vi "Configure Event Search (Serial Bus - SENT).vi"(6 "Slow Data (-1)":i32=-1, 7 "Slow ID (-1)":i32=-1, 8 "error in (no error)":errorcluster, 9 "Fast Data (0x)":string="0x", 10 "Search Operation (0: Fast Data)":i32(ring) items=["Fast Data", "Slow ID", "Slow ID and Data", "All CRC Errors", "Pulse Period Error"], 11 "VISA resource name":refnum<visa-resource-name>) -> (0 "error out":errorcluster, 3 "VISA resource name out":refnum<visa-resource-name>)   [LabVIEW 2023, in "Keysight-DSQx3014T.lvlib"]
doc: "Configures a search on a SENT serial decode signal.\n\n<b>Note:</b> SENT serial decode must be turned on and displayed in the Lister before running this VI."
uses:
  Keysight-DSQx3014T.lvlib
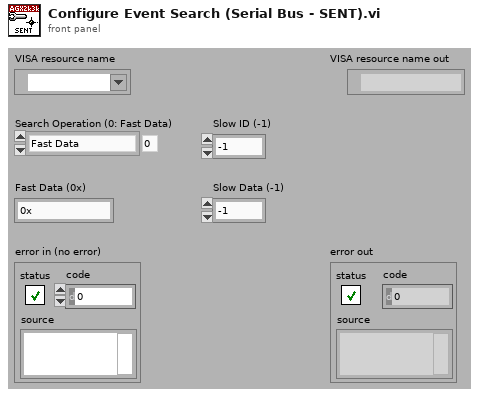
[diagram p1: front panel]
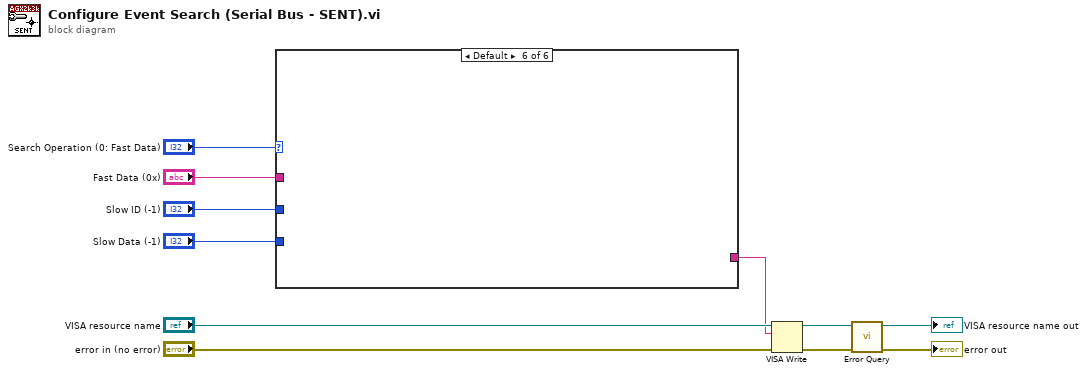
[diagram p0: block diagram]
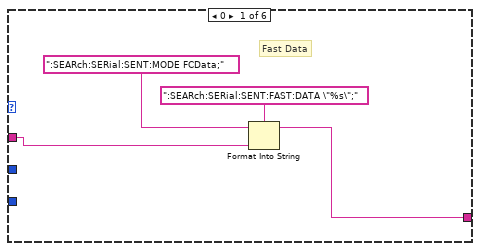
[diagram p2: hidden frame]
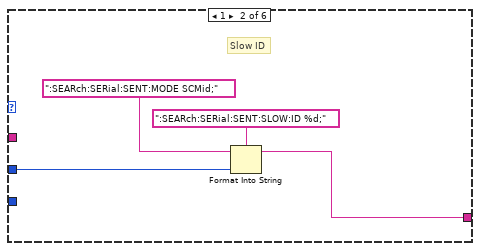
[diagram p3: hidden frame]
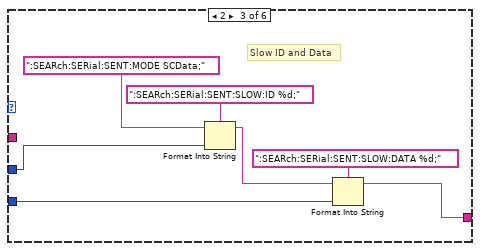
[diagram p4: hidden frame]
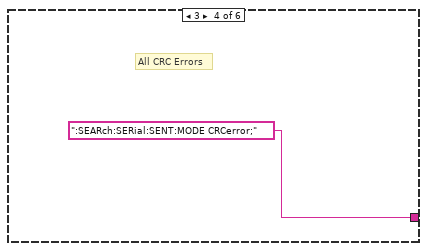
[diagram p5: hidden frame]
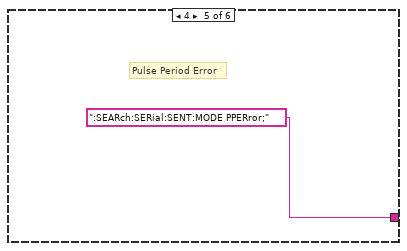
[diagram p6: hidden frame]
diagram:
  n1 = case shown="Default" "Search Operation (0: Fast Data)" {
    tunnel: "Fast Data (0x)" -> [w13 _ _ _ _ _]
    tunnel: [w12 w18 w23 ":SEARch:SERial:SENT:MODE CRCerror;" ":SEARch:SERial:SENT:MODE PPERror;" _] -> w7
    tunnel: "Slow ID (-1)" -> [_ w16 w22 _ _ _]
    tunnel: "Slow Data (-1)" -> [_ _ w20 _ _ _]
    frame 0 {
      # "Fast Data"
      n2 = Format Into String(format string=":SEARch:SERial:SENT:FAST:DATA \"%s\";", initial string=":SEARch:SERial:SENT:MODE FCData;", w13) -> (resulting string=w12:string)  [unwired: 1 in, 1 out]
    }
    frame 1 {
      # "Slow ID"
      n3 = Format Into String(format string=":SEARch:SERial:SENT:SLOW:ID %d;", initial string=":SEARch:SERial:SENT:MODE SCMid;", w16) -> (resulting string=w18:string)  [unwired: 1 in, 1 out]
    }
    frame 2 {
      # "Slow ID and Data"
      n4 = Format Into String(format string=":SEARch:SERial:SENT:SLOW:ID %d;", initial string=":SEARch:SERial:SENT:MODE SCData;", w22) -> (resulting string=w21:string)  [unwired: 1 in, 1 out]
      n5 = Format Into String(format string=":SEARch:SERial:SENT:SLOW:DATA %d;", initial string=w21, w20) -> (resulting string=w23:string)  [unwired: 1 in, 1 out]
    }
    frame 3 {
      # "All CRC Errors"
    }
    frame 4 {
      # "Pulse Period Error"
    }
    frame Default {
    }
  }
  n6 = VISA Write(VISA resource name="VISA resource name", write buffer=w7, error in (no error)="error in (no error)") -> (VISA resource name out=w4:refnum<visa-resource-name>, error out=w3:errorcluster)  [unwired: 1 out]
  n7 = call "Error Query.vi"("error in (no error)"=w3, "VISA resource name"=w4) -> ("error out"=→"error out":errorcluster, "VISA resource name out"=→"VISA resource name out":refnum<visa-resource-name>)  [unwired: 6 in, 2 out]
